vi "PathFollowing_V2.vi"() -> ()   [LabVIEW 2018]
uses:
  <vilib>/Analysis/Matrix/Datatypes/RealMatrix.ctl
  <vilib>/Utility/file.llb/Read Delimited Spreadsheet (DBL).vi
  <vilib>/Analysis/Matrix/NI_Matrix.lvlib
panel:
  out "Waveform Chart":dbl(graph)
  in  "stop":bool
  in  "Manual":bool
  in  "YPos":dbl(slide) scale=0.0..400.0
  in  "XPos":dbl(slide) scale=0.0..400.0
  out "XY Graph 2":cluster{dbl[], dbl[]}[](graph)
  in  "Number of Points":i32=200
  out "Y Output":dbl
  out "X Output":dbl
  out "robotX":dbl
  out "robotY":dbl
  in  "LookAhead":dbl=24.0
  out "myY":dbl
  out "myx":dbl
  in  "filePaths":path[](array[path])
  in  "Load Paths":bool
  out "Velocity":dbl
  in  "temp_path":T1
  in  "pathsToFollow":cluster{"Real Matrix":T1}[](array[cluster])=[{"Real Matrix"=[[64.06901469302021, 113.91217908413626, 1.0, 90.0], [111.75542049554116, 112.05260165937571, 1.0, 90.0], [142.73669523431937, 114.08839831964644, 1.0, 90.0], [145.36566303005367, 116.24536491290189, 1.0, 90.0], [147.19077325752625, 119.89009007240293, 1.0, 90.0], [151.15674341560916, 140.6038641406235, 1.0, 90.0], [153.05972300611256, 157.9433487454333, 1.0, 90.0], [155.2549588504108, 180.19410382411934, 0.0, 90.0]]}]
  out "path index":dbl
  out "Heading":dbl
  out "distance index":dbl
  out "distance":dbl
  out "intersection_y":dbl
  out "intersection_x":dbl
  in  "path":T1
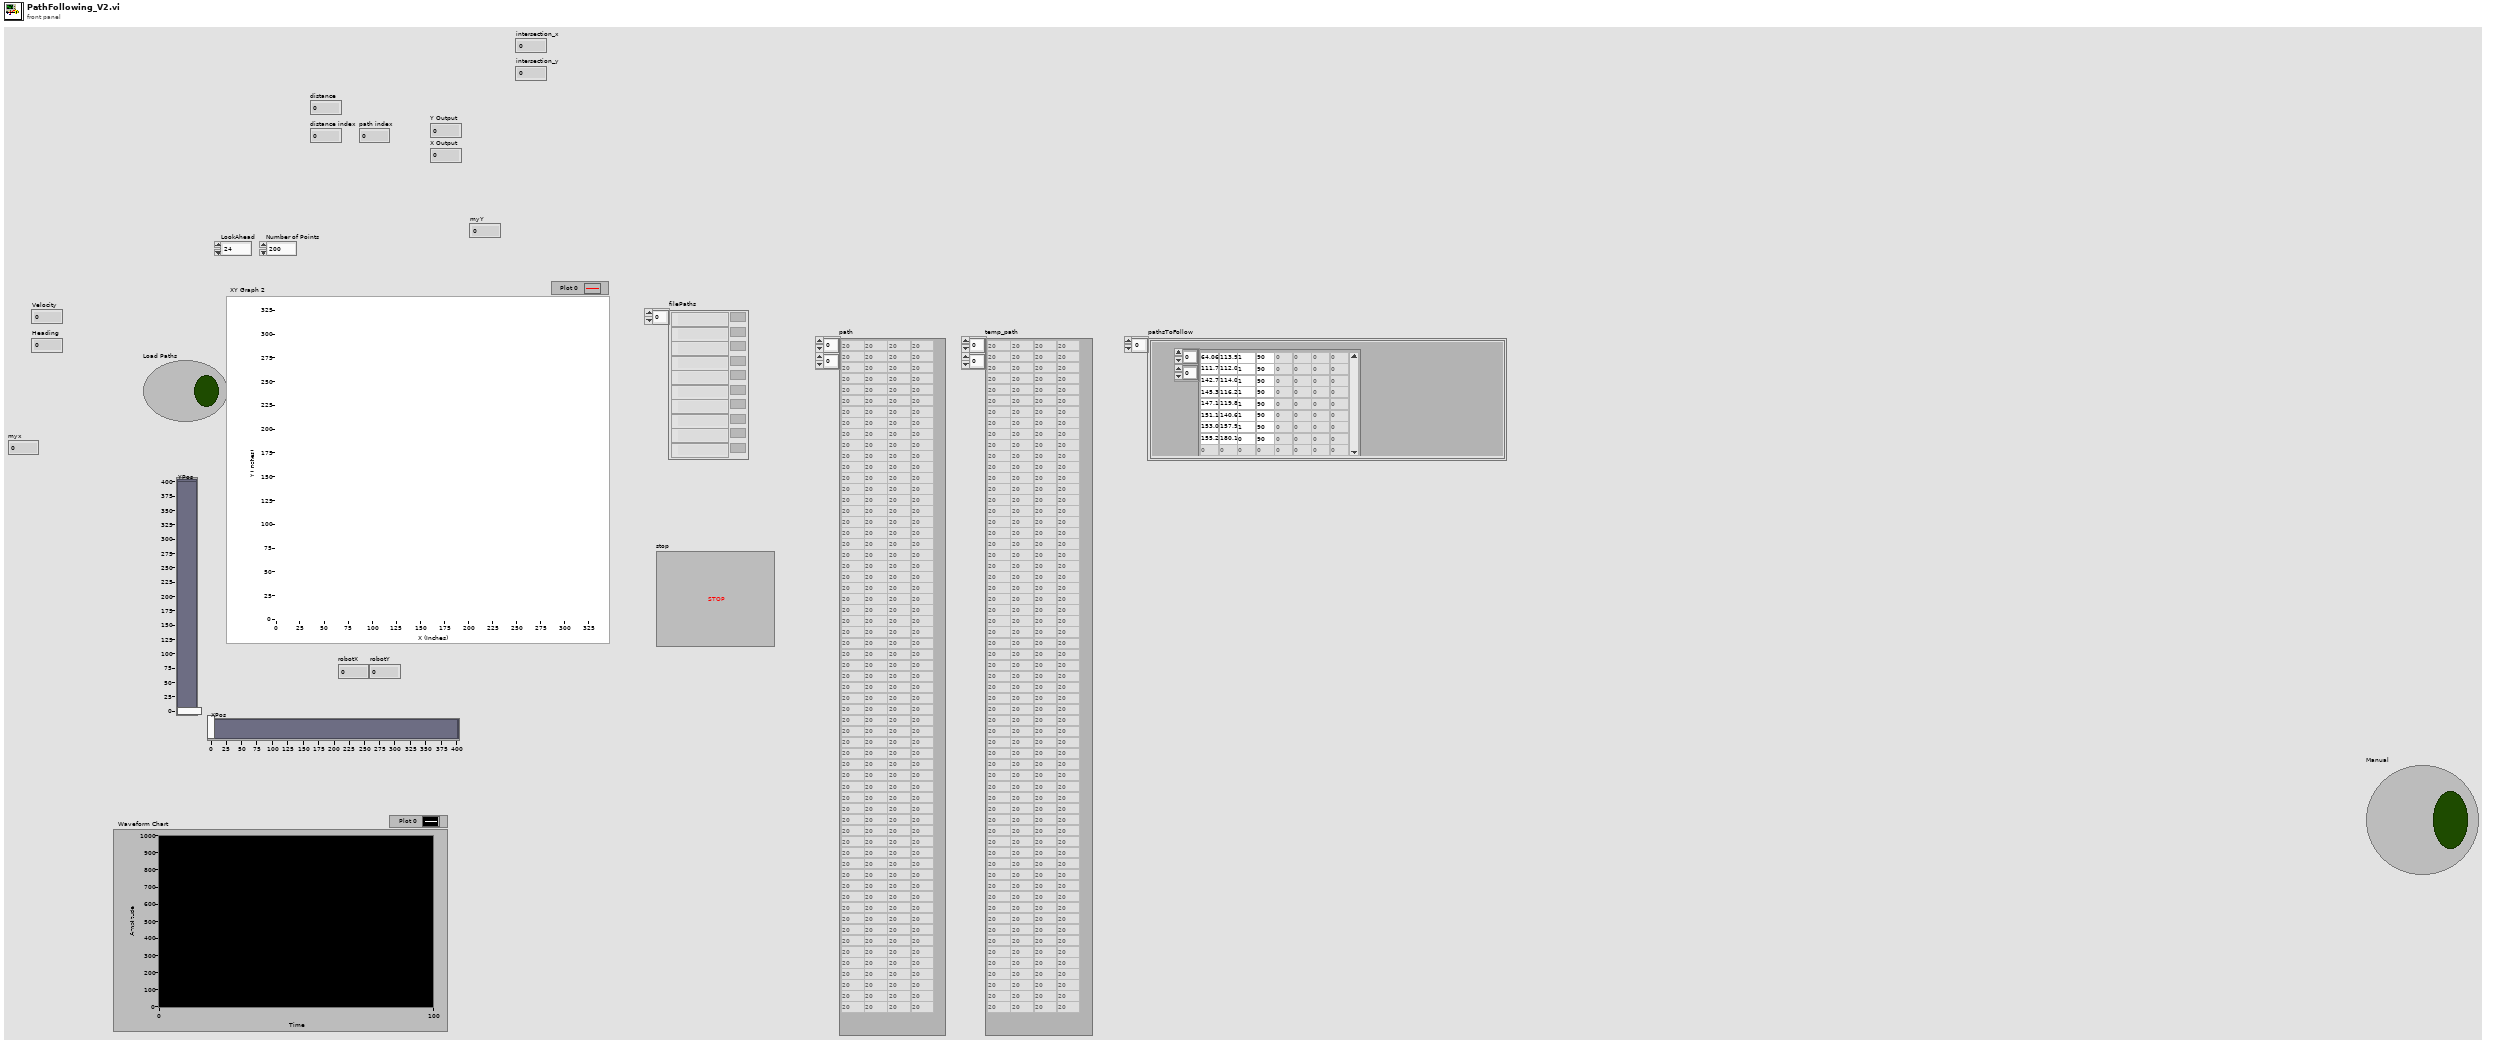
[diagram p1: front panel]
types:
  T1 = typedef "NI_Matrix.lvlib/RealMatrix.ctl" = dbl[][]
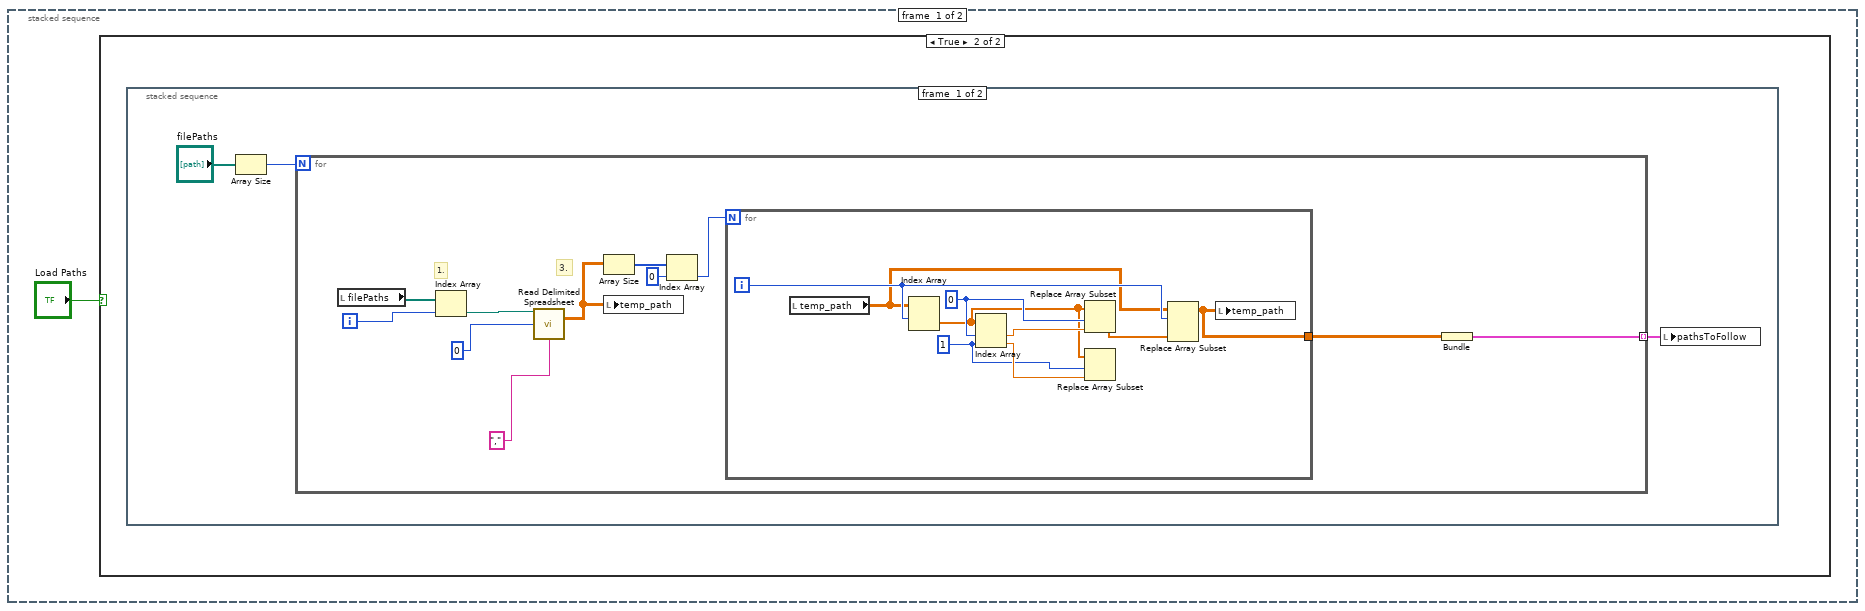
[diagram p2: hidden frame]
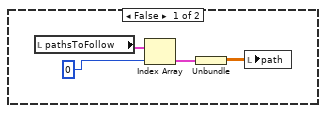
[diagram p3: hidden frame]
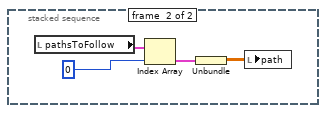
[diagram p4: hidden frame]
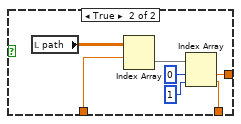
[diagram p5: hidden frame]
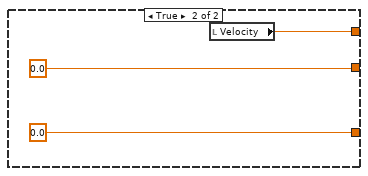
[diagram p7: hidden frame]
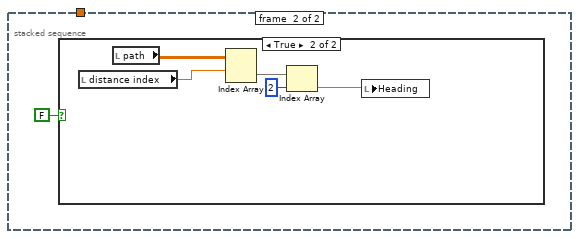
[diagram p10: hidden frame]
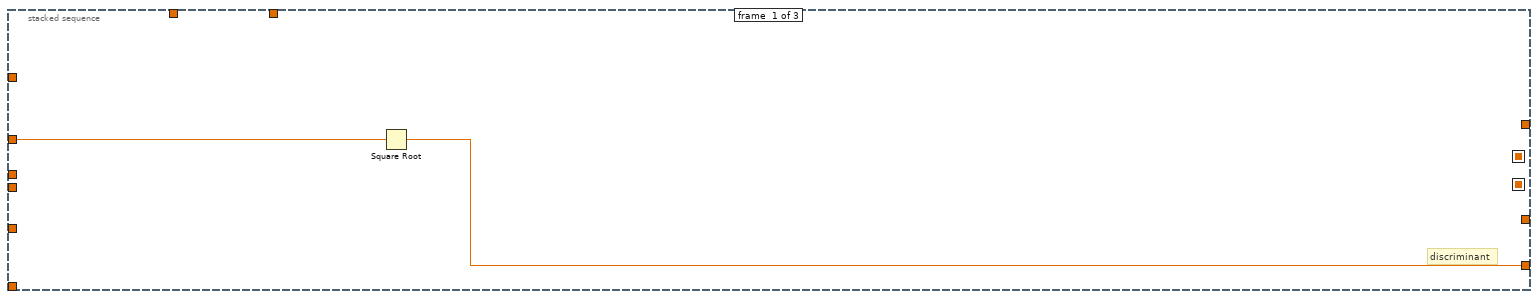
[diagram p13: hidden frame]
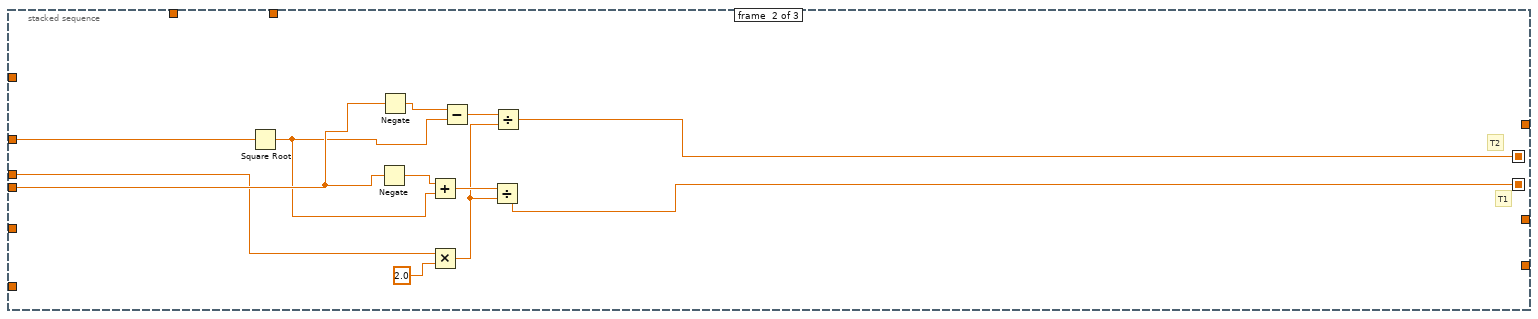
[diagram p14: hidden frame]
diagram:
  n1 = while {
    tunnel: [w11] -> _
    tunnel: [w12] -> _
    tunnel: [w13] -> _
    stop <- "stop" stop-if-true
    n2 = Not(x="Manual") -> (.not. x?=w5:bool)
    n3 = Select(t="XPos", s=w5, f="XPos") -> (s? t:f=w3:dbl)
    n4 = Select(t="YPos", s=w5, f="YPos") -> (s? t:f=w2:dbl)
    n5 = feedback #1(0.0) -> (w10:dbl)
    n6 = feedback #2(0.0) -> (w9:dbl)
    n7 = feedback #3(0.0) -> (w8:dbl)
    n8 = stacked-sequence {
      tunnel: w9 -> [_ w98]
      tunnel: [_ w72] -> _
      tunnel: w8 -> [_ w79]
      tunnel: w10 -> [_ w78]
      tunnel: [_ w75] -> w11
      tunnel: [_ w73] -> w12
      tunnel: [_ w72] -> w13
      tunnel: w3 -> [_ w50]
      tunnel: w2 -> [_ w49]
      frame #0 {
        n9 = case shown="True" "Load Paths" {
          frame False {
            n10 = local read "pathsToFollow"() -> (w20:cluster{"Real Matrix":T1}[])
            n11 = Index Array(array=w20, index=0) -> (element=w19:cluster{"Real Matrix":T1})
            n12 = Unbundle(w19) -> ("Real Matrix"=w21:T1)
            n13 = local write "path"(w21) -> ()
          }
          frame True {
            n14 = stacked-sequence {
              frame #0 {
                n15 = Array Size(array="filePaths") -> (size(s)=w24:i32)
                n16 = for {
                  N: w24 -> [_]
                  tunnel: [w26] -> w22 mode=indexing
                  i -> [w27]
                  # "3."
                  # "1."
                  n17 = local read "filePaths"() -> (w29:path[])
                  n18 = Index Array(array=w29, index=w27) -> (element=w28:path)
                  n19 = call-poly <vilib>:"Read Delimited Spreadsheet.vi"("file path (dialog if empty)"=w28, "start of read offset (chars.:0)"=0 ("mark after read (chars.)"), "delimiter (\\t)"="," ("delimiter (\\t)")) -> ("all rows"=w33:dbl[][])  [unwired: 7 in, 5 out]
                  n20 = Array Size(array=w33) -> (size(s)=w32:i32[])
                  n21 = local write "temp_path"(w33) -> ()
                  n22 = Index Array(array=w32, index=0) -> (element=w30:i32)
                  n23 = for {
                    N: w30 -> [_]
                    tunnel: [w36] -> w25
                    i -> [w44]
                    w39 = 1 ("index")
                    w43 = 0 ("index")
                    n24 = local read "temp_path"() -> (w38:T1)
                    n25 = Index Array(array=w38, index (row)=w44) -> (element=w41:dbl[])  [unwired: 1 in]
                    n26 = Index Array(array=w41, index #1=w43, index #2=w39) -> (element #1=w42:dbl, element #2=w40:dbl)
                    n27 = Replace Array Subset(array=w41, new element=w42, index=w43) -> (w37:dbl[])
                    n28 = Replace Array Subset(array=w41, new element=w40, index=w39) -> ()  [unwired: 1 out]
                    n29 = Replace Array Subset(array=w38, new element=w37, index (row)=w44) -> (w36:T1)  [unwired: 1 in]
                    n30 = local write "temp_path"(w36) -> ()
                  }
                  n31 = Bundle("temp_path"=w25) -> (w26:cluster{"temp_path":T1})  [unwired: 1 in]
                }
                n32 = local write "pathsToFollow"(w22) -> ()
              }
              frame #1 {
                n33 = local read "pathsToFollow"() -> (w47:cluster{"Real Matrix":T1}[])
                n34 = Index Array(array=w47, index=0) -> (element=w46:cluster{"Real Matrix":T1})
                n35 = Unbundle(w46) -> ("Real Matrix"=w48:T1)
                n36 = local write "path"(w48) -> ()
              }
            }
          }
        }
      }
      frame #1 {
        w71 = 2.0 ("y")
        # "y pos"
        # "x pos"
        # "X"
        # "Y"
        # "Velocity"
        # "distance index"
        # "current index"
        # "Intersection Y"
        # "Intersection X"
        # "This \"AND\" statement prevents the \"current index from being set to 0 on the last path, therefore allowing\nit to decrease in value, which is a big no no."
        # "path index"
        # "Path index"
        # "distance index"
        # "current index"
        # "distance index"
        # "current index"
        # "distance index"
        n37 = local read "pathsToFollow"() -> (w86:cluster{"Real Matrix":T1}[])
        n38 = feedback #4() -> (w87:dbl)  [unwired: 1 in]
        n39 = feedback-in #4(w78) -> ()
        n40 = local write "path index"(w78) -> ()
        n41 = Not Equal?(x=w78, y=w87) -> (x != y?=w85:bool)
        n42 = Array Size(array=w86) -> (size(s)=w82:i32)
        n43 = Less?(x=w78, y=w82) -> (x < y?=w83:bool)
        n44 = And(x=w83, y=w85) -> (x .and. y?=w84:bool)
        n45 = case shown="True" w84 {
          tunnel: w78 -> [_ w141]
          frame False {
          }
          frame True {
            n46 = local read "pathsToFollow"() -> (w142:cluster{"Real Matrix":T1}[])
            n47 = Index Array(array=w142, index=w141) -> (element=w143:cluster{"Real Matrix":T1})
            n48 = Unbundle(w143) -> ("Real Matrix"=w140:T1)
            n49 = local write "path"(w140) -> ()
          }
        }
        n50 = local read "intersection_x"() -> (w89:dbl)
        n51 = local read "intersection_y"() -> (w90:dbl)
        n52 = local read "path"() -> (w115:T1)
        n53 = Array Size(array=w115) -> (size(s)=w114:i32[])
        n54 = local read "LookAhead"() -> (w68:dbl)
        n55 = Index Array(array=w114, index=0) -> (element=w112:i32)
        n56 = local read "path"() -> (w67:T1)
        n57 = Subtract(x=w112, y=1) -> (x-y=w88:i32)
        n58 = for {
          N: w88 -> [_]
          shift-right: [w219] -> w96
          shift-left: w79 -> [w218]
          tunnel: [w217] -> w92
          tunnel: [w216] -> w91
          shift-right: [w216] -> w63
          shift-left: w90 -> [w214]
          shift-right: [w217] -> w64
          shift-left: w89 -> [w215]
          tunnel: w50 -> [w213]
          tunnel: w49 -> [w212]
          tunnel: w68 -> [w211]
          tunnel: w67 -> [w210]
          i -> [w220]
          # "Intersection Y"
          # "Intersection X"
          # "current index"
          n59 = Greater Or Equal?(x=w220, y=w218) -> (x >= y?=w221:bool)
          n60 = case shown="True" w221 {
            tunnel: w220 -> [_ w239]
            tunnel: w218 -> [w224 w238]
            tunnel: [w224 w237] -> w219
            tunnel: [w222 w236] -> w216
            tunnel: [w223 w235] -> w217
            tunnel: w215 -> [w223 w234]
            tunnel: w214 -> [w222 w233]
            tunnel: w213 -> [_ w228]
            tunnel: w212 -> [_ w227]
            tunnel: w211 -> [_ w226]
            tunnel: w210 -> [_ w225]
            frame False {
            }
            frame True {
              # "discriminant"
              # "T1"
              # "T2"
              # "current index"
              # "current index"
              # "E"
              # "L"
              # "discriminant"
              # "c"
              # "b"
              # "a"
              # "f"
              # "d"
              n61 = Add(x=w239, y=1) -> (x+y=w241:i32)
              n62 = Index Array(array=w225, index (row) #1=w239) -> (element #1=w243:dbl[])  [unwired: 3 in, 1 out]
              n63 = Index Array(array=w225, index (row) #1=w241) -> (element #1=w240:dbl[])  [unwired: 3 in, 1 out]
              n64 = Index Array(array=w243, index #1=0 ("index"), index #2=1 ("index")) -> (element #1=w250:dbl, element #2=w249:dbl)
              n65 = Index Array(array=w240, index #1=0 ("index"), index #2=1 ("index")) -> (element #1=w230:dbl, element #2=w229:dbl)
              n66 = Build Array(w250, w249) -> ()  [unwired: 1 out]
              n67 = Build Array(w230, w229) -> ()  [unwired: 1 out]
              n68 = Subtract(x=w230, y=w228) -> (x-y=w252:dbl)
              n69 = Subtract(x=w229, y=w227) -> (x-y=w251:dbl)
              n70 = Subtract(x=w250, y=w230) -> (x-y=w231:dbl)
              n71 = Subtract(x=w249, y=w229) -> (x-y=w232:dbl)
              n72 = Build Array(w231, w232) -> ()  [unwired: 1 out]
              n73 = Build Array(w252, w251) -> ()  [unwired: 1 out]
              n74 = Square(x=w226) -> (x^2=w261:dbl)
              n75 = Multiply(x=w231, y=w252) -> (x*y=w268:dbl)
              n76 = Multiply(x=w232, y=w251) -> (x*y=w267:dbl)
              n77 = Multiply(x=w252, y=w252) -> (x*y=w264:dbl)
              n78 = Multiply(x=w251, y=w251) -> (x*y=w263:dbl)
              n79 = Multiply(x=w231, y=w231) -> (x*y=w270:dbl)
              n80 = Multiply(x=w232, y=w232) -> (x*y=w269:dbl)
              n81 = Add(x=w264, y=w263) -> (x+y=w262:dbl)
              n82 = Add(x=w268, y=w267) -> (x+y=w266:dbl)
              n83 = Add(x=w270, y=w269) -> (x+y=w244:dbl)
              n84 = Subtract(x=w262, y=w261) -> (x-y=w246:dbl)
              n85 = Multiply(x=2.0, y=w266) -> (x*y=w245:dbl)
              n86 = Multiply(x=w244, y=w246) -> (x*y=w259:dbl)
              n87 = Multiply(x=w259, y=4.0) -> (x*y=w257:dbl)
              n88 = Square(x=w245) -> (x^2=w260:dbl)
              n89 = Subtract(x=w260, y=w257) -> (x-y=w247:dbl)
              n90 = Less Than 0?(x=w247) -> (x < 0?=w248:bool)
              n91 = case shown="False" w248 {
                tunnel: w247 -> [w284 _]
                tunnel: w245 -> [w283 _]
                tunnel: w244 -> [w282 _]
                tunnel: w239 -> [w281 _]
                tunnel: w238 -> [w279 w361]
                tunnel: [w280 w361] -> w237
                tunnel: [w278 w359] -> w236
                tunnel: [w277 w360] -> w235
                tunnel: w234 -> [w276 w360]
                tunnel: w233 -> [w275 w359]
                tunnel: w232 -> [w274 _]
                tunnel: w231 -> [w273 _]
                tunnel: w230 -> [w272 _]
                tunnel: w229 -> [w271 _]
                frame False {
                  n92 = stacked-sequence {
                    seq-local: [_ w288 _] -> [_ _ w303]
                    seq-local: [_ w287 _] -> [_ _ w304]
                    tunnel: w284 -> [w286 w290 _]
                    tunnel: w283 -> [_ w292 _]
                    tunnel: w282 -> [_ w291 _]
                    tunnel: w281 -> [_ _ w314]
                    tunnel: w279 -> [_ _ w315]
                    tunnel: [_ _ w318] -> w280
                    tunnel: [_ _ w308] -> w277
                    tunnel: [_ _ w307] -> w278
                    tunnel: w276 -> [_ _ w306]
                    tunnel: w275 -> [_ _ w305]
                    tunnel: [w285 _ _] -> _
                    tunnel: w274 -> [_ _ w302]
                    tunnel: w273 -> [_ _ w301]
                    tunnel: w272 -> [_ _ w299]
                    tunnel: w271 -> [_ _ w300]
                    frame #0 {
                      # "discriminant"
                      n93 = Square Root(x=w286) -> (sqrt(x)=w285:dbl)
                    }
                    frame #1 {
                      # "T1"
                      # "T2"
                      n94 = Square Root(x=w290) -> (sqrt(x)=w289:dbl)
                      n95 = Negate(x=w292) -> (-x=w295:dbl)
                      n96 = Negate(x=w292) -> (-x=w298:dbl)
                      n97 = Add(x=w295, y=w289) -> (x+y=w294:dbl)
                      n98 = Multiply(x=w291, y=2.0) -> (x*y=w293:dbl)
                      n99 = Subtract(x=w298, y=w289) -> (x-y=w297:dbl)
                      n100 = Divide(x=w294, y=w293) -> (x/y=w287:dbl)
                      n101 = Divide(x=w297, y=w293) -> (x/y=w288:dbl)
                    }
                    frame #2 {
                      n102 = Greater Or Equal To 0?(x=w304) -> (x >= 0?=w317:bool)
                      n103 = Less Or Equal?(x=w304, y=1.0) -> (x <= y?=w316:bool)
                      n104 = And(x=w317, y=w316) -> (x .and. y?=w311:bool)
                      n105 = case shown="True" w311 {
                        tunnel: w304 -> [_ w337]
                        tunnel: [w324 w335] -> w312
                        tunnel: [w323 w334] -> w309
                        tunnel: w314 -> [_ w332]
                        tunnel: w315 -> [w325 w331]
                        tunnel: [w325 w330] -> w313
                        tunnel: w306 -> [w324 _]
                        tunnel: w305 -> [w323 _]
                        tunnel: w302 -> [_ w329]
                        tunnel: w301 -> [_ w328]
                        tunnel: w299 -> [_ w327]
                        tunnel: w300 -> [_ w326]
                        frame False {
                        }
                        frame True {
                          # "E"
                          # "current index"
                          # "intersection y"
                          # "intersection x"
                          n106 = Multiply(x=w337, y=w329) -> (x*y=w336:dbl)
                          n107 = Multiply(x=w337, y=w328) -> (x*y=w338:dbl)
                          n108 = Greater?(x=w332, y=w331) -> (0:w333:bool)
                          n109 = Add(x=w327, y=w338) -> (x+y=w335:dbl)
                          n110 = Add(x=w326, y=w336) -> (x+y=w334:dbl)
                          n111 = case shown="True" w333 {
                            tunnel: w332 -> [_ w340]
                            tunnel: [w339 w340] -> w330
                            tunnel: w331 -> [w339 _]
                            frame False {
                            }
                            frame True {
                            }
                          }
                        }
                      }
                      n112 = Greater Or Equal To 0?(x=w303) -> (x >= 0?=w320:bool)
                      n113 = Less Or Equal?(x=w303, y=1.0) -> (x <= y?=w321:bool)
                      n114 = And(x=w320, y=w321) -> (x .and. y?=w322:bool)
                      n115 = case shown="True" w322 {
                        tunnel: w303 -> [_ w355]
                        tunnel: [w343 w353] -> w308
                        tunnel: [w341 w352] -> w307
                        tunnel: w312 -> [w343 _]
                        tunnel: w314 -> [_ w350]
                        tunnel: w313 -> [w342 w349]
                        tunnel: [w342 w348] -> w318
                        tunnel: w309 -> [w341 _]
                        tunnel: w302 -> [_ w347]
                        tunnel: w301 -> [_ w346]
                        tunnel: w300 -> [_ w345]
                        tunnel: w299 -> [_ w344]
                        frame False {
                        }
                        frame True {
                          # "current index"
                          # "intersection y"
                          # "intersection x"
                          n116 = Multiply(x=w355, y=w347) -> (x*y=w354:dbl)
                          n117 = Multiply(x=w355, y=w346) -> (x*y=w356:dbl)
                          n118 = Greater?(x=w350, y=w349) -> (0:w351:bool)
                          n119 = Add(x=w344, y=w356) -> (x+y=w353:dbl)
                          n120 = Add(x=w345, y=w354) -> (x+y=w352:dbl)
                          n121 = case shown="True" w351 {
                            tunnel: w350 -> [_ w358]
                            tunnel: [w357 w358] -> w348
                            tunnel: w349 -> [w357 _]
                            frame False {
                            }
                            frame True {
                            }
                          }
                        }
                      }
                    }
                  }
                }
                frame True {
                }
              }
            }
          }
        }
        n122 = stacked-sequence {
          tunnel: [w158 _] -> w97
          tunnel: w98 -> [w159 _]
          tunnel: w50 -> [w155 _]
          tunnel: w49 -> [w154 _]
          frame #0 {
            n123 = local read "path"() -> (w163:T1)
            n124 = Array Size(array=w163) -> (size(s)=w162:i32[])
            n125 = local read "path"() -> (w157:T1)
            n126 = Index Array(array=w162, index=0) -> (element=w160:i32)
            n127 = for {
              N: w160 -> [_]
              shift-right: [w173] -> w158
              shift-left: w159 -> [w172]
              tunnel: w155 -> [w170]
              tunnel: w154 -> [w169]
              shift-right: [w168] -> _
              shift-left: 1000000000.0 -> [w165]
              shift-right: [w167] -> _
              shift-left: _ -> [w166]
              tunnel: w157 -> [w164]
              i -> [w174]
              # "distance"
              # "current index"
              n128 = case shown="True" TRUE {
                tunnel: w174 -> [_ w186]
                tunnel: [w177 w185] -> w173
                tunnel: w172 -> [w177 w184]
                tunnel: w170 -> [_ w183]
                tunnel: w169 -> [_ w182]
                tunnel: [w175 w181] -> w168
                tunnel: [w176 w180] -> w167
                tunnel: w166 -> [w176 _]
                tunnel: w165 -> [w175 w178]
                tunnel: w164 -> [_ w179]
                frame False {
                }
                frame True {
                  n129 = Index Array(array=w179, index (row)=w186) -> (element=w198:dbl[])  [unwired: 1 in]
                  n130 = Index Array(array=w198, index #1=0 ("index"), index #2=1 ("index")) -> (element #1=w194:dbl, element #2=w195:dbl)
                  n131 = Subtract(x=w195, y=w182) -> (x-y=w192:dbl)
                  n132 = Subtract(x=w194, y=w183) -> (x-y=w193:dbl)
                  n133 = Square(x=w192) -> (x^2=w191:dbl)
                  n134 = Square(x=w193) -> (x^2=w190:dbl)
                  n135 = Add(x=w191, y=w190) -> (x+y=w189:dbl)
                  n136 = Square Root(x=w189) -> (sqrt(x)=w187:dbl)
                  n137 = Less?(x=w187, y=w178) -> (x < y?=w188:bool)
                  n138 = case shown="True" w188 {
                    tunnel: w187 -> [w199 w203]
                    tunnel: w186 -> [w200 w202]
                    tunnel: [w201 w202] -> w185
                    tunnel: w184 -> [w201 _]
                    tunnel: [w199 w203] -> w181
                    tunnel: [w200 w202] -> w180
                    frame False {
                    }
                    frame True {
                      # "distance"
                      # "distance index"
                    }
                  }
                  "Waveform Chart" <- w178
                }
              }
            }
          }
          frame #1 {
            n139 = case shown="True" FALSE {
              frame False {
              }
              frame True {
                n140 = local read "distance index"() -> (w208:dbl)
                n141 = local read "path"() -> (w209:T1)
                n142 = Index Array(array=w209, index (row)=w208) -> (element=w207:dbl[])  [unwired: 1 in]
                n143 = Index Array(array=w207, index=2) -> (element=w205:dbl)
                n144 = local write "Heading"(w205) -> ()
              }
            }
          }
        }
        n145 = local write "intersection_x"(w64) -> ()
        n146 = local write "intersection_y"(w63) -> ()
        n147 = local read "path"() -> (w105:T1)
        n148 = Array Size(array=w105) -> (size(s)=w106:i32[])
        n149 = Index Array(array=w106, index=0) -> (element=w104:i32)
        n150 = local read "pathsToFollow"() -> (w81:cluster{"Real Matrix":T1}[])
        n151 = Add(x=w97, y=1.0) -> (x+y=w100:dbl)
        n152 = Equal?(x=w104, y=w100) -> (x = y?=w95:bool)
        n153 = Build Array(w50, w50) -> (w127:dbl[])
        n154 = Build Array(w49, w49) -> (w126:dbl[])
        n155 = Select(t=1.0, s=w95, f=0.0) -> (s? t:f=w101:dbl)
        n156 = Array Size(array=w81) -> (size(s)=w80:i32)
        n157 = Add(x=w101, y=w78) -> (x+y=w72:dbl)
        n158 = Build Array(w92, w92) -> (w110:dbl[])
        n159 = Build Array(w91, w91) -> (w109:dbl[])
        n160 = local read "path"() -> (w124:T1)
        n161 = Bundle(w127, w126) -> (w116:cluster{dbl[], dbl[]})  [unwired: 1 in]
        n162 = Less?(x=w72, y=w80) -> (x < y?=w93:bool)
        n163 = And(x=w95, y=w93) -> (x .and. y?=w94:bool)
        n164 = Array Size(array=w124) -> (size(s)=w121:i32[])
        n165 = case shown="False" w94 {
          tunnel: [w147 0.0 ("distance index")] -> w73
          tunnel: w97 -> [w147 _]
          tunnel: w96 -> [w148 _]
          tunnel: [w148 0.0 ("currentIndex")] -> w75
          tunnel: [w144 w151] -> w74
          frame False {
            n166 = local read "path"() -> (w146:T1)
            n167 = Index Array(array=w146, index (row) #1=w147, index (col) #1=2 ("disabled index (col)"), index (row) #2=w147, index (col) #2=3 ("disabled index (col)")) -> (element #1=w144:dbl, element #2=w145:dbl)
            n168 = local write "Heading"(w145) -> ()
            n169 = local write "Velocity"(w144) -> ()
          }
          frame True {
            n170 = local read "Velocity"() -> (w151:dbl)
          }
        }
        n171 = Bundle(w110, w109) -> (w108:cluster{dbl[], dbl[]})  [unwired: 1 in]
        n172 = Index Array(array=w121, index=0) -> (element=w119:i32)
        n173 = local read "path"() -> (w70:T1)
        n174 = for {
          N: w119 -> [_]
          tunnel: [w364] -> w123 mode=indexing
          tunnel: [w363] -> w122 mode=indexing
          tunnel: w70 -> [w362]
          i -> [w368]
          n175 = Index Array(array=w362, index (row)=w368) -> (element=w367:dbl[])  [unwired: 1 in]
          n176 = Index Array(array=w367, index #1=0 ("index"), index #2=1 ("index")) -> (element #1=w364:dbl, element #2=w363:dbl)
        }
        n177 = for {
          N: "Number of Points" -> [_]
          tunnel: "Number of Points" -> [w380]
          tunnel: [w373] -> w128 mode=indexing
          tunnel: [w372] -> w129 mode=indexing
          tunnel: w49 -> [w371]
          tunnel: w50 -> [w370]
          tunnel: "LookAhead" -> [w369]
          i -> [w382]
          n178 = Multiply(x=6.283185307179586, y=w382) -> (x*y=w381:dbl)
          n179 = Divide(x=w381, y=w380) -> (x/y=w378:dbl)
          n180 = Sine & Cosine(0:w378) -> (1:w377:dbl, 2:w376:dbl)
          n181 = Multiply(x=w377, y=w369) -> (x*y=w375:dbl)
          n182 = Multiply(x=w376, y=w369) -> (x*y=w374:dbl)
          n183 = Add(x=w375, y=w370) -> (x+y=w373:dbl)
          n184 = Add(x=w374, y=w371) -> (x+y=w372:dbl)
        }
        n185 = Bundle(w123, w122) -> (w117:cluster{dbl[], dbl[]})  [unwired: 1 in]
        n186 = Bundle(w128, w129) -> (w118:cluster{dbl[], dbl[]})  [unwired: 1 in]
        n187 = Build Array(w108, w116, w118, w117) -> (→"XY Graph 2":cluster{dbl[], dbl[]}[])
        n188 = case shown="False" FALSE {
          tunnel: w75 -> [_ w135]
          tunnel: [w131 w134] -> w62
          tunnel: [w132 w133] -> w61
          frame False {
            n189 = local read "intersection_x"() -> (w132:dbl)
            n190 = local read "intersection_y"() -> (w131:dbl)
          }
          frame True {
            n191 = local read "path"() -> (w139:T1)
            n192 = Index Array(array=w139, index (row)=w135) -> (element=w138:dbl[])  [unwired: 1 in]
            n193 = Index Array(array=w138, index #1=0 ("index"), index #2=1 ("index")) -> (element #1=w133:dbl, element #2=w134:dbl)
          }
        }
        n194 = Subtract(x=w61, y=w50) -> (x-y=w77:dbl)
        n195 = Subtract(x=w62, y=w49) -> (x-y=w76:dbl)
        n196 = Inverse Tangent (2 Input)(1:w77, 2:w76) -> (0:w53:dbl)
        n197 = Add(x=w53, y=1.57) -> (x+y=w51:dbl)
        n198 = Sine & Cosine(0:w51) -> (1:w60:dbl, 2:w59:dbl)
        n199 = Multiply(x=w74, y=w60) -> (x*y=w66:dbl)
        "Y Output" <- w66
        n200 = Multiply(x=w59, y=w74) -> (x*y=w65:dbl)
        "X Output" <- w65
        n201 = Divide(x=w66, y=w71) -> (x/y=w57:dbl)
        n202 = Divide(x=w65, y=w71) -> (x/y=w56:dbl)
        n203 = Negate(x=w57) -> (-x=→"myx":dbl)
        n204 = Negate(x=w56) -> (-x=→"myY":dbl)
        "robotX" <- w50
        "robotY" <- w49
      }
    }
    n205 = feedback-in #1(w13) -> ()
    n206 = feedback-in #2(w12) -> ()
    n207 = feedback-in #3(w11) -> ()
  }
